vi "compute_mandelbrot_set.vi"(7 "max iter":i32=100, 10 "y axis":T1={"samples"=1000, "end"=1.0, "start"=-1.0}, 11 "x axis":T1={"samples"=1000, "end"=1.0, "start"=-2.0}) -> (2 "render time":dbl, 3 "fractal set":i32[][](graph))   [LabVIEW 2019, in "Mandelbrot.lvlib"]
uses:
  Mandelbrot.lvlib
  axis_info.ctl
  <vilib>/Analysis/1siggen.llb/Ramp Pattern by Samples.vi
  <vilib>/Analysis/NI_AALBase.lvlib
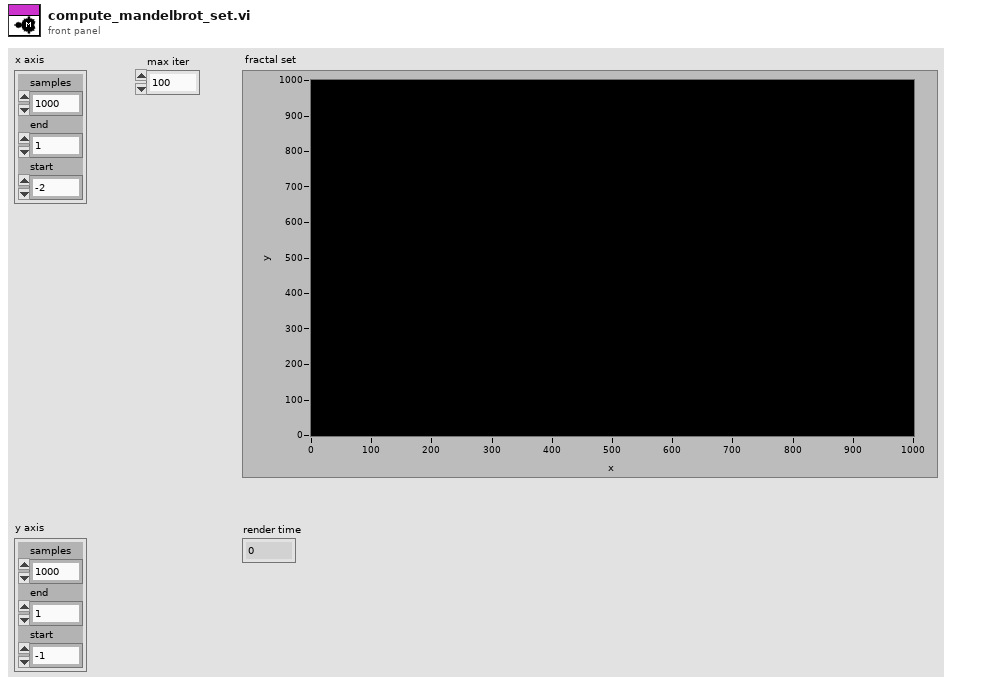
[diagram p1: front panel]
types:
  T1 = typedef "Mandelbrot.lvlib/axis_info.ctl" = cluster{"samples":u32, "end":dbl, "start":dbl}
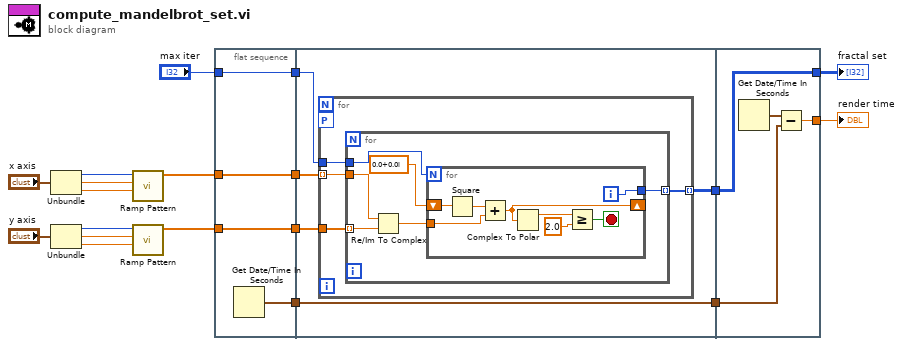
[diagram p0: block diagram]
diagram:
  n1 = Unbundle("x axis") -> ("samples"=w18:u32, "end"=w17:dbl, "start"=w16:dbl)
  n2 = Unbundle("y axis") -> ("samples"=w14:u32, "end"=w13:dbl, "start"=w12:dbl)
  n3 = call-poly <vilib>:"Ramp Pattern.vi"("start"=w16, "end"=w17, "samples"=w18) -> ("Ramp Pattern"=w10:dbl[])  [unwired: 7 in, 1 out]
  n4 = call-poly <vilib>:"Ramp Pattern.vi"("start"=w12, "end"=w13, "samples"=w14) -> ("Ramp Pattern"=w9:dbl[])  [unwired: 7 in, 1 out]
  n5 = flat-sequence {
    tunnel: w9 -> [w21]
    tunnel: w10 -> [w22]
    tunnel: "max iter" -> [w23]
    tunnel: [w23] -> w6
    tunnel: [w22] -> w5
    tunnel: [w21] -> w4
    tunnel: [w20] -> w3
    tunnel: [w25] -> w7
    tunnel: w6 -> [w28]
    tunnel: w5 -> [w27]
    tunnel: w4 -> [w26]
    tunnel: w3 -> [w24]
    tunnel: [w24] -> w2
    tunnel: [w50] -> w8
    tunnel: w7 -> [w50]
    tunnel: w2 -> [w48]
    tunnel: [w47] -> w1
    frame #0 {
      n6 = Get Date/Time In Seconds() -> (seconds since 1Jan1904=w20:timestamp)
    }
    frame #1 {
      n7 = for {
        tunnel: w28 -> [w32]
        tunnel: w27 -> [w31] mode=indexing
        tunnel: w26 -> [w30]
        tunnel: [w29] -> w25 mode=indexing
        workers-P: _ -> [_]
        n8 = for {
          tunnel: w32 -> [w38]
          tunnel: w31 -> [w37]
          tunnel: w30 -> [w36] mode=indexing
          tunnel: [w34] -> w29 mode=indexing
          n9 = Re/Im To Complex(1:w36, 2:w37) -> (0:w33:cdb)
          n10 = for {
            N: w38 -> [_]
            shift-right: [w41] -> _
            shift-left: cdb 0.0+0.0i ("x + iy") -> [w46]
            tunnel: w33 -> [w44]
            tunnel: [w39] -> w34
            i -> [w39]
            stop <- w40 stop-if-true
            n11 = Square(x=w46) -> (x^2=w45:cdb)
            n12 = Add(x=w45, y=w44) -> (x+y=w41:cdb)
            n13 = Complex To Polar(r * e^(i*theta)=w41) -> (r=w43:dbl)  [unwired: 1 out]
            n14 = Greater Or Equal?(x=w43, y=2.0) -> (x >= y?=w40:bool)
          }
        }
      }
    }
    frame #2 {
      n15 = Get Date/Time In Seconds() -> (seconds since 1Jan1904=w49:timestamp)
      n16 = Subtract(x=w49, y=w48) -> (x-y=w47:dbl)
    }
  }
  "fractal set" <- w8
  "render time" <- w1
